vi "Circular_trajectory_of_tip_with_time_close_loop_final.vi"() -> ()   [LabVIEW 2019]
uses:
  <vilib>/FPGAPlugInAG/sbRIO-9629/niLvFpga_Open_sbRIO-9629.vi
  <vilib>/rvi/interface/common/dynamic/niFpgaDynamicAddResources.vi
  <vilib>/Utility/error.llb/Error Cluster From Error Code.vi
  <vilib>/rvi/errors/niLvFpgaAdjustHostInterfaceError.vi
  <vilib>/FPGAPlugInAG/Dynamic/niLvFpga_Close_Dynamic.vi
  <vilib>/rvi/interface/nirviOpenFPGA/nirviOpenFPGA.xnode
  FPGA Bitfiles/fcmsinglesection_FPGATarget_CloseLoopMotorTu_eGt+d+EV+VE.lvbitx
  Close_Loop_Motor_Tune.vi
  <vilib>/rvi/interface/nirviReadWriteControl/nirviReadWriteControl.xnode
  <vilib>/rvi/interface/nirviCloseFPGA/nirviCloseFPGA.xnode
  NiFpgaLv.dll
  <vilib>/rvi/interface/Simulation/niFpgaSimulationCallBeginRW.vi
panel:
  in  "Ki":dbl
  out "alpha_e":dbl
  out "L_v_e":dbl
  in  "Motor3_KP":sgl
  in  "Motor2_KP":sgl
  in  "Motor1_KP":sgl
  out "logical OR":bool
  in  "Kp":dbl
  out "Error":dbl[](array[numeric])
  out "Current Tip Position":dbl[](array[numeric])
  out "data out":string
  in  "radius":dbl=0.2
  in  "Degree Steps":dbl
  out "Tip Position":dbl[](array[numeric])
  out "theta1":dbl
  out "theta2":dbl
  out "theta3":dbl
  out "L_v":dbl
  out "alpha":dbl
  in  "Start Time":dbl
  in  "End Time":dbl
  out "t":dbl[](array[numeric])
  out "Error":errorcluster
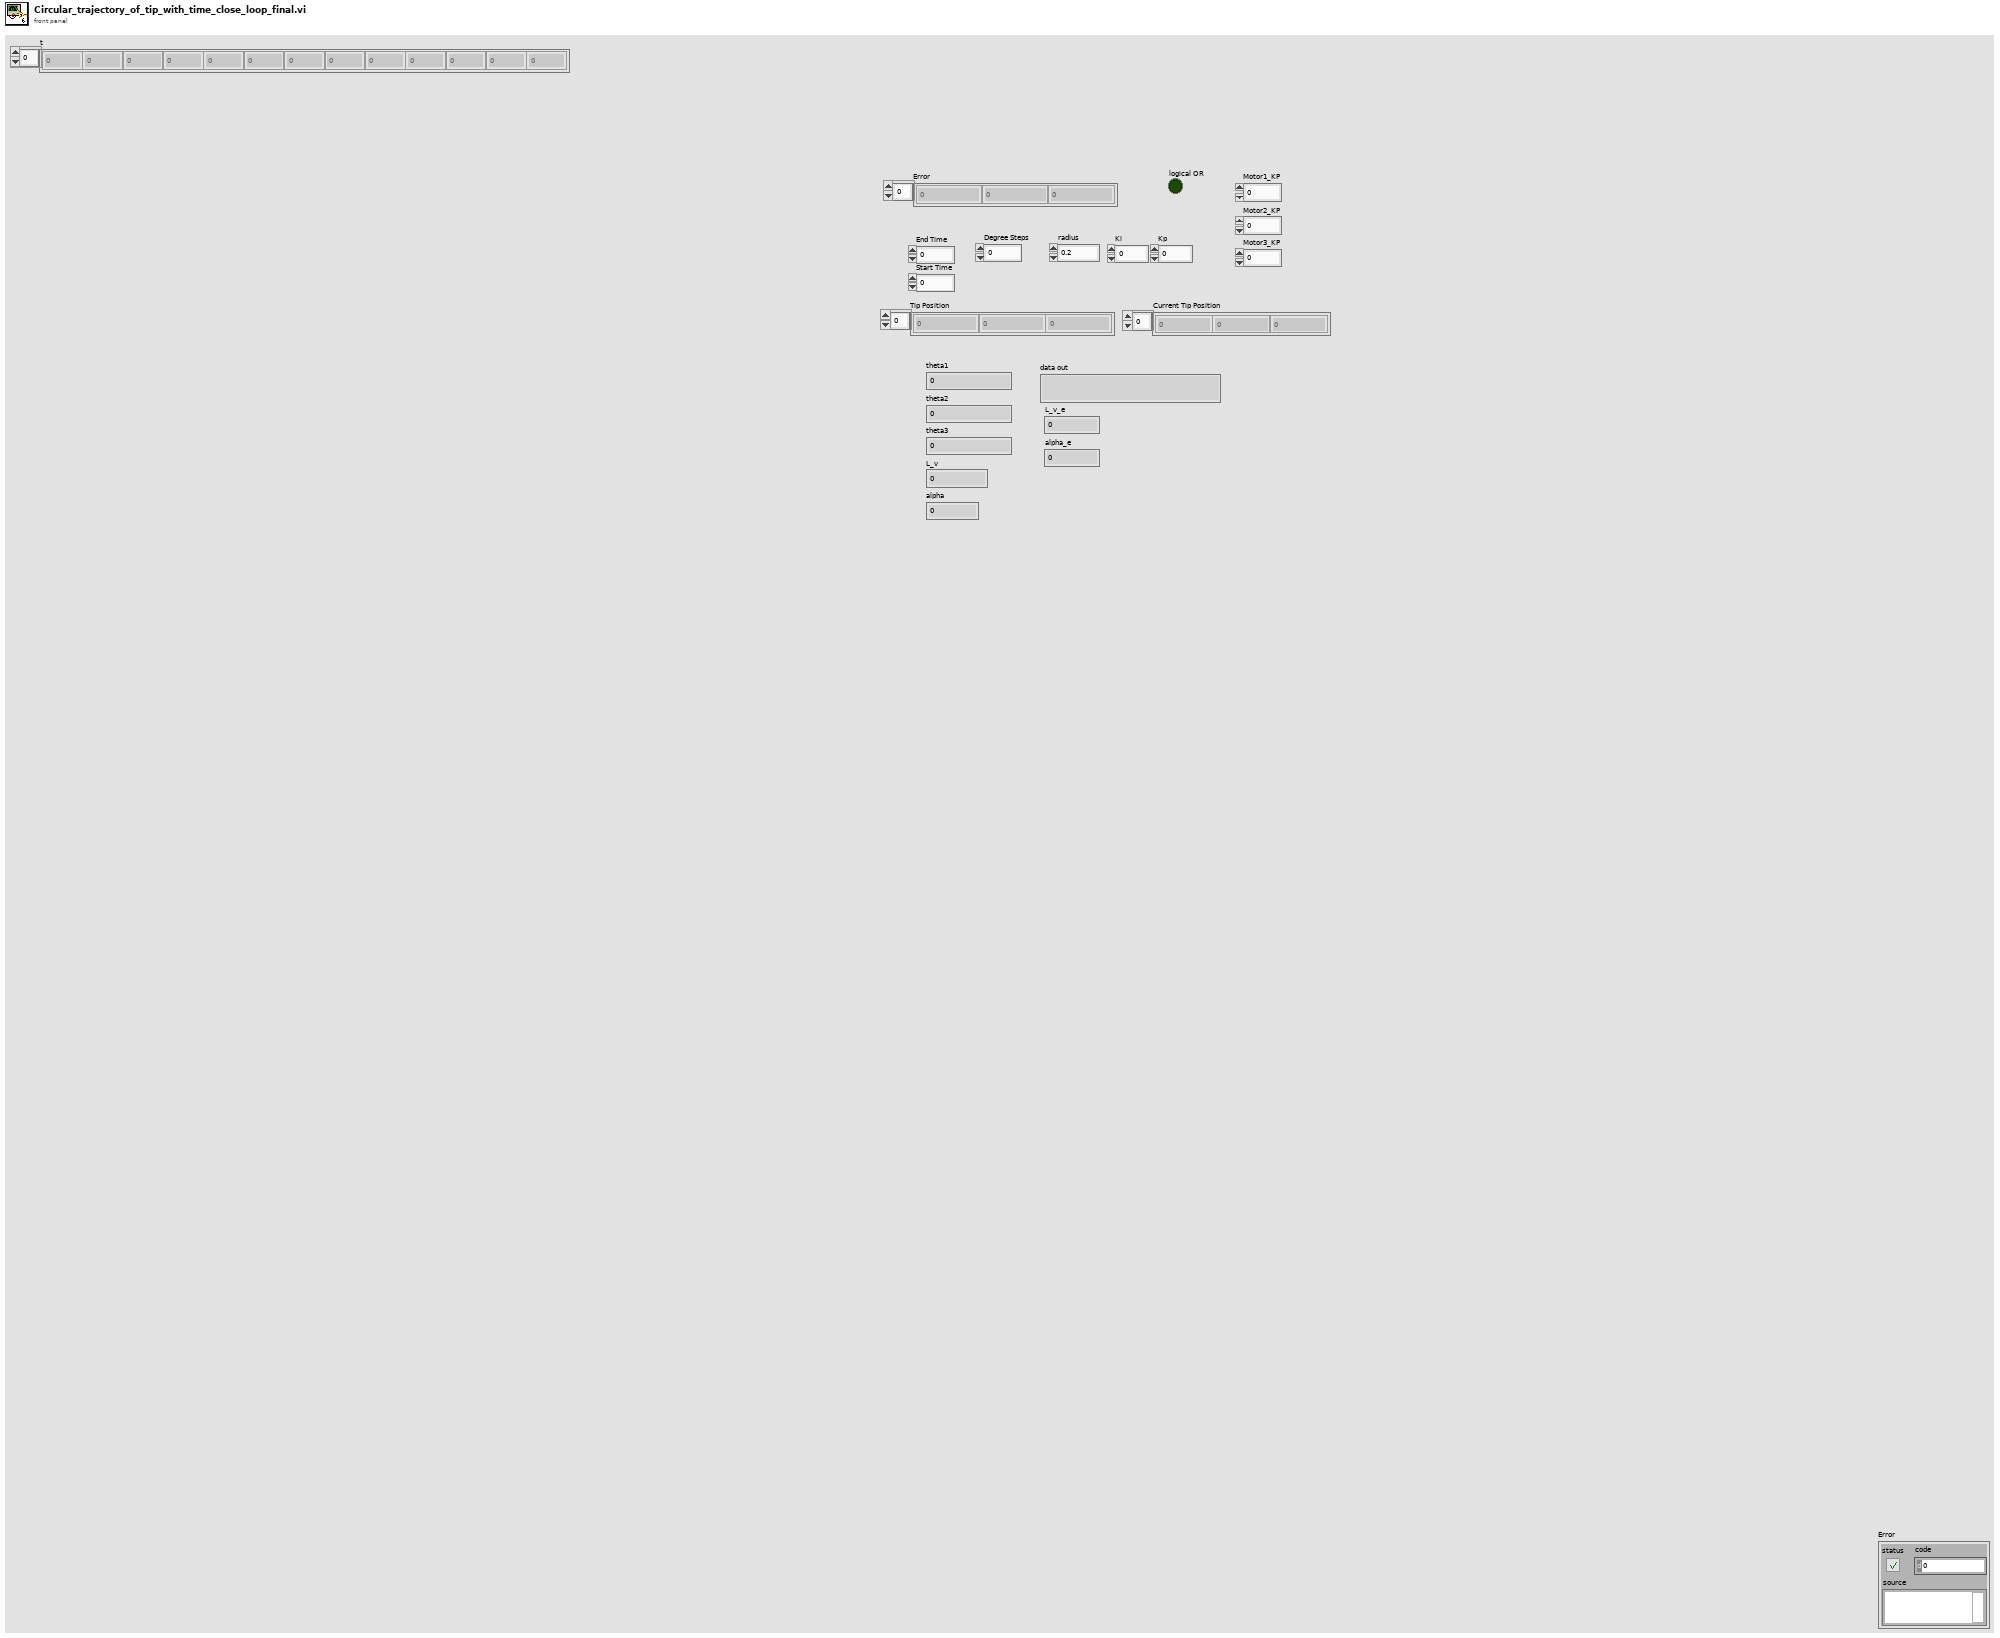
[diagram p1: front panel]
types:
  T1 = enum16{"open", "open or create", "create or replace", "create", "open (read-only)"}
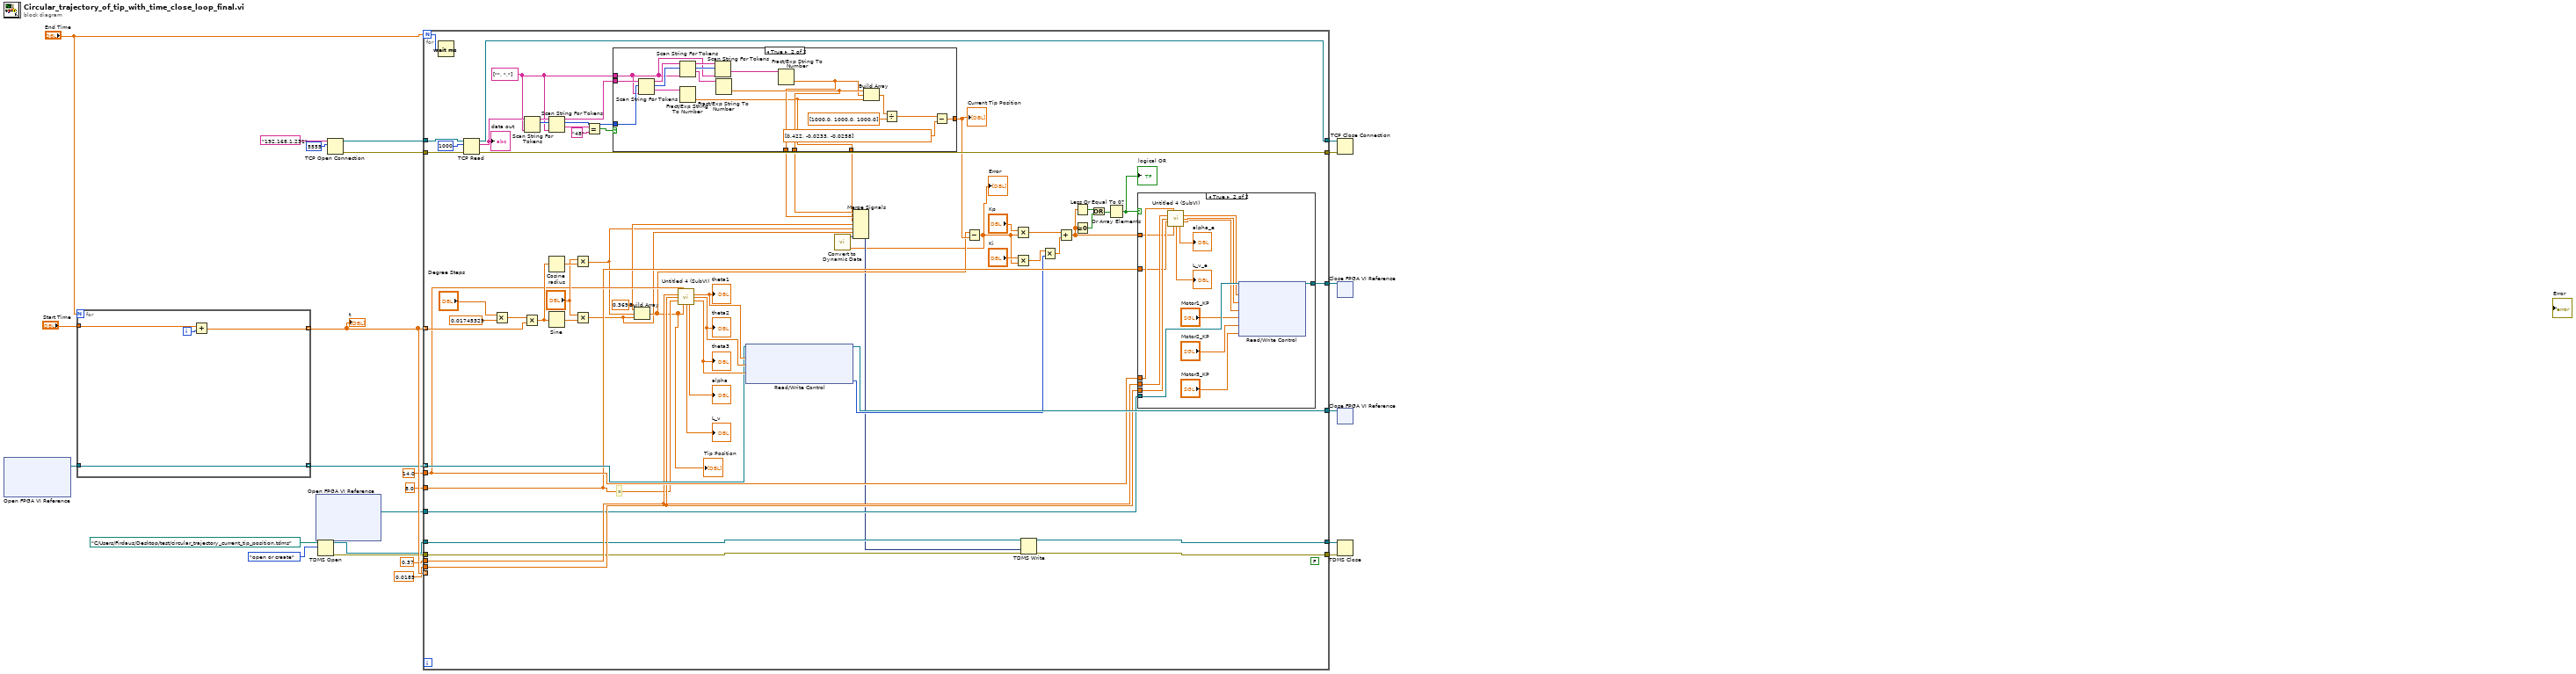
[diagram p0: block diagram]
diagram:
  n1 = xnode "Open FPGA VI Reference"() -> ("FPGA VI Reference Out"=w18:refnum<k20>)  [unwired: 2 in, 1 out]
  n2 = for {
    N: "End Time" -> [_]
    tunnel: "Start Time" -> [w27]
    tunnel: [w26] -> w23 mode=indexing
    tunnel: w18 -> [w25]
    tunnel: [w25] -> w17 mode=indexing
    i -> [w28]
    n3 = Add(x=w27, y=w28) -> (x+y=w26:dbl)
  }
  "t" <- w23
  n4 = xnode "Open FPGA VI Reference"() -> ("FPGA VI Reference Out"=w7:refnum<k20>)  [unwired: 2 in, 1 out]
  n5 = TDMS Open(10:T1."open or create" ("operation (0:open)"), 11:path "C:/Users/Firdaus/Desktop/test/circular_trajectory_current_tip_position.tdms" ("file path")) -> (0:w5:errorcluster, 3:w6:refnum<k34>)  [unwired: 5 in]
  n6 = TCP Open Connection(address="192.168.1.231", remote port or service name=u16 5555) -> (connection ID=w15:refnum<k5>, error out=w14:errorcluster)  [unwired: 3 in]
  n7 = for {
    N: "End Time" -> [w50]
    tunnel: w23 -> [w81] mode=indexing
    tunnel: w23 -> [_] mode=indexing
    tunnel: 0.37 ("Length of the FCM (m)") -> [w55]
    tunnel: 0.0185 ("Radius of disk (m)") -> [w54]
    tunnel: 8.0 ("Number of Disks") -> [w53]
    tunnel: 14.0 ("Radius of motor pulley\n (mm)") -> [w56]
    tunnel: w17 -> [w83] mode=indexing
    tunnel: [w82] -> w16
    tunnel: w15 -> [w75]
    tunnel: w14 -> [w74]
    tunnel: [w73] -> w13
    tunnel: [w72] -> w12
    tunnel: w7 -> [w52]
    tunnel: [w51] -> w9
    tunnel: w6 -> [w43]
    tunnel: w5 -> [w42]
    tunnel: [w41] -> w4
    tunnel: [w40] -> w3
    (unwired) FALSE
    w62 = string[] ["", ","] ("delimiters (\\s,\\t,\\r,\\n)")
    w33 = 0.369
    # "x"
    n8 = Wait (ms)(milliseconds to wait=w50) -> ()  [unwired: 1 out]
    n9 = TCP Read(connection ID=w75, bytes to read=1000, error in (no error)=w74) -> (connection ID out=w72:refnum<k5>, data out=w66:string, error out=w73:errorcluster)  [unwired: 2 in]
    "data out" <- w66
    n10 = Multiply(x="Degree Steps", y=0.01745329) -> (x*y=w77:dbl)
    n11 = Multiply(x=w77, y=w81) -> (x*y=w80:dbl)
    n12 = Scan String For Tokens(6:w62, 9:w66) -> (2:w68:i32, 3:w69:string)  [unwired: 4 in, 2 out]
    n13 = Scan String For Tokens(6:w62, 8:w68, 9:w69) -> (1:w70:string, 2:w63:i32, 3:w64:string)  [unwired: 3 in, 1 out]
    n14 = Cosine(x=w80) -> (cos(x)=w90:dbl)
    n15 = Sine(x=w80) -> (sin(x)=w89:dbl)
    n16 = Multiply(x="radius", y=w90) -> (x*y=w32:dbl)
    n17 = Multiply(x="radius", y=w89) -> (x*y=w31:dbl)
    n18 = Equal?(x=w70, y="48") -> (x = y?=w65:bool)
    n19 = case shown="True" w65 {
      tunnel: [_ w112] -> w39
      tunnel: w64 -> [_ w111]
      tunnel: w63 -> [_ w110]
      tunnel: w62 -> [_ w109]
      tunnel: [_ w108] -> w37
      tunnel: [_ w107] -> w36
      tunnel: [_ w106] -> w35
      frame False {
      }
      frame True {
        n20 = Scan String For Tokens(6:w109, 8:w110, 9:w111) -> (1:w119:string, 2:w121:i32, 3:w123:string)  [unwired: 3 in, 1 out]
        n21 = Scan String For Tokens(6:w109, 8:w121, 9:w123) -> (1:w118:string, 2:w120:i32, 3:w122:string)  [unwired: 3 in, 1 out]
        n22 = Fract/Exp String To Number(string=w119) -> (number=w106:dbl)  [unwired: 3 in, 1 out]
        n23 = Scan String For Tokens(6:w109, 8:w120, 9:w122) -> (1:w117:string)  [unwired: 3 in, 3 out]
        n24 = Fract/Exp String To Number(string=w118) -> (number=w108:dbl)  [unwired: 3 in, 1 out]
        n25 = Fract/Exp String To Number(string=w117) -> (number=w107:dbl)  [unwired: 3 in, 1 out]
        n26 = Build Array(w108, w107, w106) -> (w116:dbl[])
        n27 = Divide(x=w116, y=dbl[] [1000.0, 1000.0, 1000.0]) -> (x/y=w114:dbl[])
        n28 = Subtract(x=w114, y=dbl[] [0.422, -0.0233, -0.0258]) -> (x-y=w112:dbl[])
      }
    }
    "Current Tip Position" <- w39
    n29 = Build Array(w33, w32, w31) -> (w38:dbl[])
    "Tip Position" <- w38
    n30 = call "Untitled 4 (SubVI).vi"("Radius of motor pulley\n (mm)"=w56, "Length of the FCM (m)"=w55, "Radius of disk (m)"=w54, "Number of Disks"=w53, "Tip position Input"=w38) -> ("theta1"=w86:dbl, "theta2"=w85:dbl, "theta3"=w84:dbl, "L_v"=→"L_v":dbl, "alpha"=→"alpha":dbl)  [unwired: 2 in, 4 out]
    "theta1" <- w86
    "theta2" <- w85
    "theta3" <- w84
    n31 = xnode "Read/Write Control"("FPGA VI Reference In"=w83, "desired angle"=w86, "desired angle 2"=w85, "desired angle 3"=w84) -> ("FPGA VI Reference Out"=w82:refnum<k20>, "Loop time (position) 1 motor side _e"=w47:u32)  [unwired: 1 in, 1 out]
    n32 = Subtract(x=w38, y=w39) -> (x-y=w30:dbl[])
    "Error" <- w30
    n33 = call "Convert to Dynamic Data"("Array"=w30) -> ("Dynamic Data Type"=w29:dynamicdata)  [unwired: 3 in]
    n34 = Merge Signals(w37, w36, w35, w33, w32, w31, w29) -> (w34:dynamicdata)
    n35 = Multiply(x="Kp", y=w30) -> (x*y=w46:dbl[])
    n36 = Multiply(x="Ki", y=w30) -> (x*y=w48:dbl[])
    n37 = TDMS Write(0:w43, 9:w34, 11:w42) -> (4:w40:refnum<k34>, 15:w41:errorcluster)  [unwired: 3 in, 2 out]
    n38 = Multiply(x=w48, y=w47) -> (x*y=w45:dbl[])
    n39 = Add(x=w46, y=w45) -> (x+y=w44:dbl[])
    n40 = Less Or Equal To 0?(x=w44) -> (x <= 0?=w60:bool[])
    n41 = Greater Or Equal To 0?(x=w44) -> (x >= 0?=w59:bool[])
    n42 = Or(x=w60, y=w59) -> (x .or. y?=w58:bool[])
    n43 = Or Array Elements(Boolean array=w58) -> (logical OR=w57:bool)
    "logical OR" <- w57
    n44 = case shown="True" w57 {
      tunnel: w56 -> [_ w105]
      tunnel: w55 -> [_ w104]
      tunnel: w54 -> [_ w103]
      tunnel: w53 -> [_ w102]
      tunnel: w44 -> [_ w101]
      tunnel: w52 -> [_ w100]
      tunnel: [_ w99] -> w51
      frame False {
      }
      frame True {
        n45 = call "Untitled 4 (SubVI).vi"("Radius of motor pulley\n (mm)"=w105, "Length of the FCM (m)"=w104, "Radius of disk (m)"=w103, "Number of Disks"=w102, "Tip position Input"=w101) -> ("theta1"=w98:dbl, "theta2"=w97:dbl, "theta3"=w96:dbl, "L_v"=→"L_v_e":dbl, "alpha"=→"alpha_e":dbl)  [unwired: 2 in, 4 out]
        n46 = xnode "Read/Write Control"("FPGA VI Reference In"=w100, "desired angle (error)"=w98, "desired angle 2(error)"=w97, "desired angle 3(error)"=w96, "Motor1_KP"="Motor1_KP", "Motor2_KP"="Motor2_KP", "Motor3_KP"="Motor3_KP") -> ("FPGA VI Reference Out"=w99:refnum<k20>)  [unwired: 1 in, 1 out]
      }
    }
  }
  n47 = TCP Close Connection(connection ID=w12, error in (no error)=w13) -> ()  [unwired: 1 in, 2 out]
  n48 = xnode "Close FPGA VI Reference"("FPGA VI Reference In"=w9) -> ()  [unwired: 1 in, 1 out]
  n49 = xnode "Close FPGA VI Reference"("FPGA VI Reference In"=w16) -> ()  [unwired: 1 in, 1 out]
  n50 = TDMS Close(8:w4, 11:w3) -> ()  [unwired: 2 out]
